vi "8P_Process.vi"(0 "All samples in":sgl[][](array[numeric]), 1 "8HP Ch No":i16[](array[numeric]), 2 "Analysis info Index":i32[](array[numeric]), 3 "Sampling Rate":dbl) -> ()   [LabVIEW 2020]
uses:
  Globals/Meas_global.vi
  Sub_vis/Upload Data.ctl
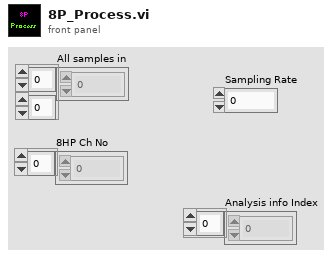
[diagram p1: front panel]
types:
  T1 = typedef "Upload Data.ctl" = enum16{"Voltage Array", "Time Trace Cluster"}
  T2 = typedef "Analysis_info_cluster.ctl" = cluster{"Colour":u32, "Inst type":T3, "Inst name":string, "Symbol":string, "Code name":string, "Extra Info":string, "Inst Array":T4, "Extra Titles":string[], "Extra Values":string[], "U":dbl, "u^2":dbl, "u^3":dbl, "u^4":dbl, "Skew_u":dbl, "Kurt_u":dbl, "Sd Error in Mean":dbl, "% u'/U":dbl, "X":dbl, "Y":dbl, "Z":dbl, "Timescale integral Estimate":dbl, "Sd Error in Variance":dbl, "Calib File":path, "Calib Constants":dbl[], "Output Position":bool, "Stats":enum16{"None", "Basic", "Full"}, "Av Sampling Rate":dbl, "Av No of Samples":dbl, "Total Meas Time (s)":dbl, "ADAM Ch Name":string, "Max value":dbl, "Min value":dbl, "Req Sample Rate Hz":dbl, "Sync Delay Time (s)":dbl, "Ch No":i16, "Device":string, "Use Latest Calib":bool, "Port":string, "Metadata Ch Names":string[], "Metadata Ch Values":string[], "Label":string}
  T3 = typedef "Inst_type.ctl" = enum16{"Raw voltage", "Raw with zero offsetting", "Propeller anemometer", "Pressure Transducer", "Pitot-static tube", "Hot wire", "Cross wire 1", "Cross wire 2", "Generic Linear", "Generic Polynomial", "Generic BackPoly", "Fast FID", "Thermocouple", "Cold wire", "Pulsed Wire", "LDA Vel", "LDA Tran time", "LDA Arr time", "Microphone"}
  T4 = typedef "Instrument_Array.ctl" = enum16{"PWA", "LDA", "Analogue"}
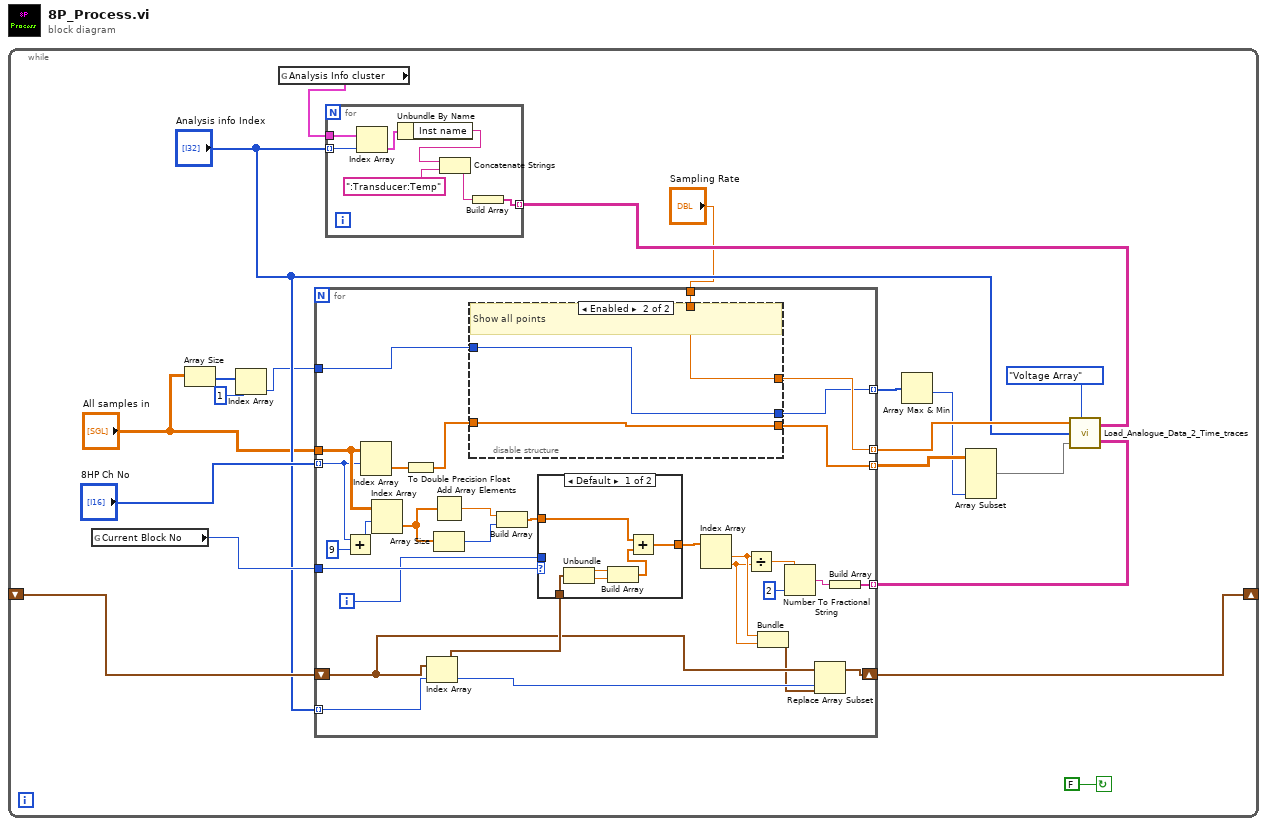
[diagram p0: block diagram]
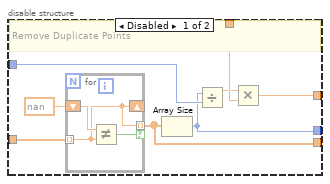
[diagram p2: hidden frame]
diagram:
  n1 = while {
    shift-right: [w12] -> _
    shift-left: _ -> [w13]
    stop <- FALSE continue-if-true
    n2 = global read "Meas_global.vi" "Current Block No"() -> (w15:i32)
    n3 = Array Size(array="All samples in") -> (size(s)=w9:i32[])
    n4 = Index Array(array=w9, index=1) -> (element=w3:i32)
    n5 = global read "Meas_global.vi" "Analysis Info cluster"() -> (w20:T2[])
    n6 = for {
      tunnel: "8HP Ch No" -> [w45] mode=indexing
      tunnel: "All samples in" -> [w48]
      tunnel: [w22] -> w7 mode=indexing
      tunnel: [w24] -> w18 mode=indexing
      tunnel: w15 -> [w43]
      tunnel: [w35] -> w19 mode=indexing
      tunnel: "Sampling Rate" -> [w25]
      shift-right: [w27] -> w12
      shift-left: w13 -> [w29]
      tunnel: "Analysis info Index" -> [w31] mode=indexing
      tunnel: w3 -> [w23]
      tunnel: [w21] -> w5 mode=indexing
      i -> [w42]
      n7 = Add(x=w45, y=9) -> (x+y=w46:i32)
      n8 = Index Array(array=w48, index (row)=w45) -> (element=w49:sgl[])  [unwired: 1 in]
      n9 = Index Array(array=w48, index (row)=w46) -> (element=w44:sgl[])  [unwired: 1 in]
      n10 = To Double Precision Float(number=w49) -> (double precision float=w26:dbl[])
      n11 = Index Array(array=w29, index=w31) -> (element=w30:cluster{"Numeric":sgl, "Numeric":sgl})
      n12 = Add Array Elements(numeric array=w44) -> (sum=w40:sgl)
      n13 = Array Size(array=w44) -> (size(s)=w39:i32)
      n14 = disable-structure shown="Enabled" {
        disable-tunnel: w26 -> [w57 w63]
        disable-tunnel: w25 -> [w56 w62]
        disable-tunnel: [w55 w62] -> w24
        disable-tunnel: w23 -> [w54 w61]
        disable-tunnel: [w53 w63] -> w22
        disable-tunnel: [w52 w61] -> w21
        frame Disabled {
          # "Remove Duplicate Points"
          n15 = for {
            shift-right: [w59] -> _
            shift-left: nan -> [w60]
            tunnel: w57 -> [w59] mode=indexing
            tunnel: [w59] -> w53 mode=indexing if=w58
            n16 = Not Equal?(x=w60, y=w59) -> (x != y?=w58:bool)
          }
          n17 = Array Size(array=w53) -> (size(s)=w52:i32)
          n18 = Divide(x=w52, y=w54) -> (x/y=w50:dbl)
          n19 = Multiply(x=w50, y=w56) -> (x*y=w55:dbl)
        }
        frame Enabled {
          # "Show all points"
        }
      }
      n20 = Build Array(w40, w39) -> (w41:sgl[])
      n21 = case shown="Default" w43 {
        tunnel: w42 -> [_ _]
        tunnel: w41 -> [w69 w70]
        tunnel: [w68 w70] -> w34
        tunnel: w30 -> [w67 _]
        frame Default {
          n22 = Unbundle(w67) -> ("Numeric"=w66:sgl, "Numeric"=w65:sgl)
          n23 = Build Array(w66, w65) -> (w64:sgl[])
          n24 = Add(x=w69, y=w64) -> (x+y=w68:sgl[])
        }
        frame 1 {
        }
      }
      n25 = Index Array(array=w34) -> (element #1=w33:sgl, element #2=w32:sgl)  [unwired: 2 in]
      n26 = Divide(x=w33, y=w32) -> (x/y=w37:sgl)
      n27 = Bundle("Numeric"=w33, "Numeric"=w32) -> (w28:cluster{"Numeric":sgl, "Numeric":sgl})  [unwired: 1 in]
      n28 = Number To Fractional String(number=w37, precision (6)=i16 2) -> (F-format string=w36:string)  [unwired: 2 in]
      n29 = Replace Array Subset(array=w29, new element=w28, index=w31) -> (w27:cluster{"Numeric":sgl, "Numeric":sgl}[])
      n30 = Build Array(w36) -> (w35:string[])
    }
    n31 = for {
      tunnel: w20 -> [w77]
      tunnel: "Analysis info Index" -> [w76] mode=indexing
      tunnel: [w71] -> w17 mode=indexing
      n32 = Index Array(array=w77, index=w76) -> (element=w75:T2)
      n33 = Unbundle By Name(w75) -> ("Inst name"=w74:string)
      n34 = Concatenate Strings(w74, ":Transducer:Temp" ("string")) -> (w72:string)
      n35 = Build Array(w72) -> (w71:string[])
    }
    n36 = Array Max & Min(array=w5) -> (min value=w4:i32)  [unwired: 3 out]
    n37 = Array Subset(array=w7, length (col)=w4) -> (w6:dbl[][])  [unwired: 3 in]
    n38 = call "Load_Analogue_Data_2_Time_traces.vi"("Sampling Rate (Hz)"=w18, "Mode"=Upload_Data."Voltage Array", "Index"="Analysis info Index", "Voltage Array"=w6, "Metadata Names"=w17, "Metadata Values"=w19) -> ()  [unwired: 1 in]
  }
